vi "CleanUp.vi"(0 "object in":refnum<class "RedState.lvclass">, 5 "Error In":errorcluster) -> (14 "object out":refnum<class "RedState.lvclass">, 19 "Error Out":errorcluster)   [LabVIEW 2024, in "RedState.lvclass"]
uses:
  RedState.lvclass
  RedState.lvclass/RedState.ctl
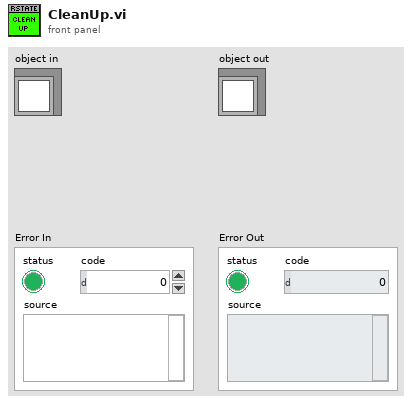
[diagram p1: front panel]
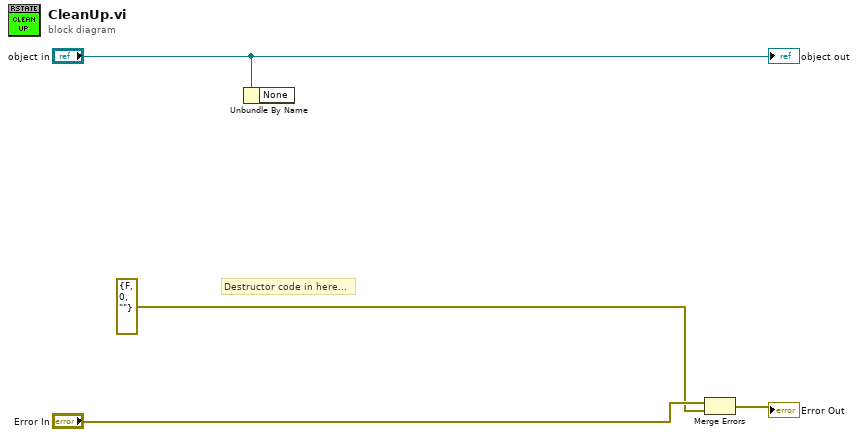
[diagram p0: block diagram]
diagram:
  # "Destructor code in here..."
  n1 = Unbundle By Name("object in") -> ()  [unwired: 1 out]
  n2 = Merge Errors("Error In", errorcluster {"status"=FALSE, "code"=0, "source"=""} ("error in (no error)")) -> (→"Error Out":errorcluster)
  "object out" <- "object in"
